vi "goto xyz.vi"(8 "error in (no error)":errorcluster, 9 "z":i16, 10 "y":i16, 11 "x":i16) -> (0 "error out":errorcluster)   [LabVIEW 2015, in "SCANalone4x64.lvlib"]
doc: "__declspec(dllimport) void __stdcall goto_xyz(short x, short y, short z);"
uses:
  <userlib>/SCANalone4x64/SCANalone4x64.lvlib
  <userlib>/SCANalone4x64/SCANalone4x64.dll
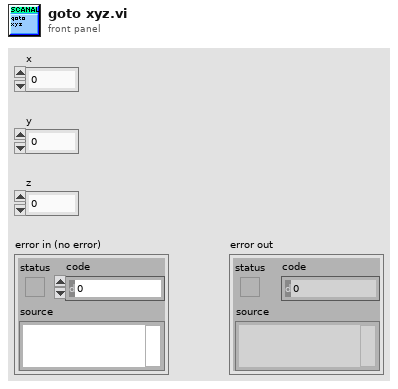
[diagram p1: front panel]
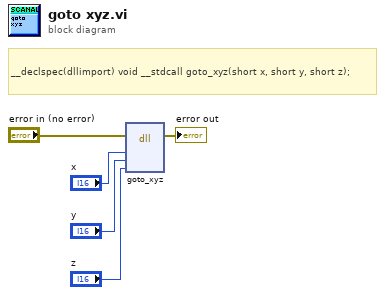
[diagram p0: block diagram]
diagram:
  # "__declspec(dllimport) void __stdcall goto_xyz(short x, short y, short z);"
  n1 = dll-call lib="C:/Program Files/National Instruments/LabVIEW 2015/user.lib/SCANalone4x64/SCANalone4x64.*" fn="goto_xyz"(error in="error in (no error)", "x"="x", "y"="y", "z"="z") -> (error out=→"error out":errorcluster)  [unwired: 6 in, 1 out]
